vi "Out of Bounds.vi"(7 "error source vi name":string, 8 "error in (no error)":errorcluster, 9 "size":u64 format="%d bytes", 10 "offset":u64 format="%d bytes", 11 "Pointer in":refnum<class "Pointer.lvclass">) -> (0 "error out":errorcluster, 3 "Pointer out":refnum<class "Pointer.lvclass">)   [LabVIEW 2020, in "Memory Manager.lvlib" / "Pointer.lvclass"]
uses:
  Pointer.lvclass
  Errors.ctl
  VIs/Write Numeric Scalar to Source (Base10 U64).vi
  Static Errors.lvlib
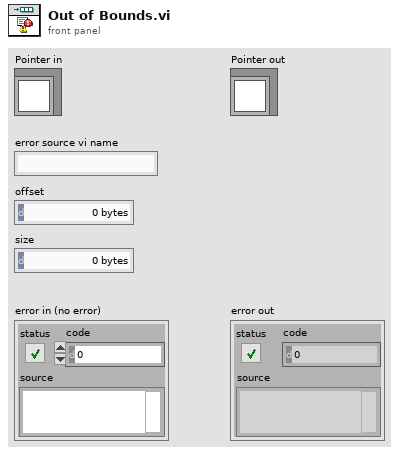
[diagram p1: front panel]
types:
  T1 = typedef "Memory Manager.lvlib/Pointer.lvclass/Errors.ctl" = enum16{"No Error", "Null Pointer", "Out of Bounds", "Buffer Underflow", "Size Mismatch", "Zone"}
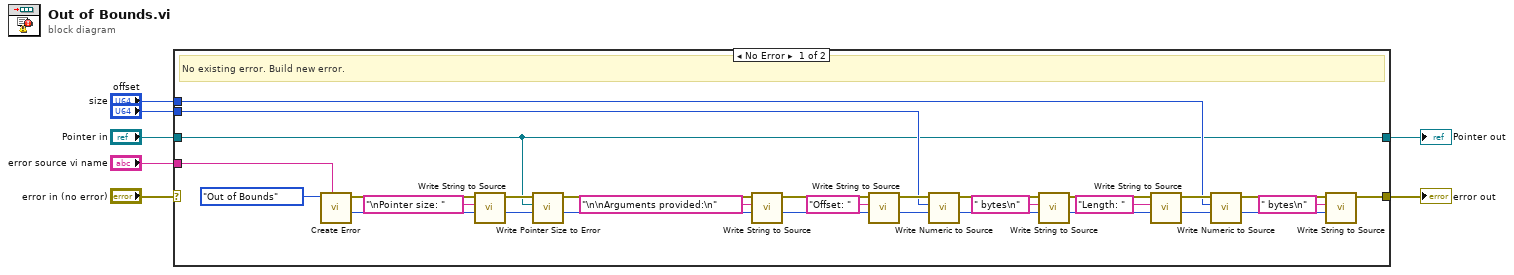
[diagram p0: block diagram]
diagram:
  n1 = case shown="No Error" "error in (no error)" {
    selector: "error in (no error)" -> [_ w39]
    tunnel: [w16 w39] -> w4
    tunnel: "offset" -> [w28 _]
    tunnel: "error source vi name" -> [w32 _]
    tunnel: "Pointer in" -> [w8 w38]
    tunnel: [w8 w38] -> w2
    tunnel: "size" -> [w15 _]
    frame No Error {
      # "No existing error. Build new error."
      n2 = call "Create Error.vi"("source vi name"=w32, "error"=Errors."Out of Bounds") -> ("new offset"=w34:i32, "error out"=w35:errorcluster)  [unwired: 8 in]
      n3 = call "Write String to Source.vi"("offset"=w34, "string"="\nPointer size: ", "error in"=w35) -> ("new offset"=w36:i32, "error out"=w9:errorcluster)  [unwired: 7 in]
      n4 = call "Write Pointer Size to Error.vi"("offset"=w36, "Pointer"=w8, "error in"=w9) -> ("new offset"=w12:i32, "error out"=w10:errorcluster)  [unwired: 7 in]
      n5 = call "Write String to Source.vi"("offset"=w12, "string"="\n\nArguments provided:\n", "error in"=w10) -> ("new offset"=w13:i32, "error out"=w14:errorcluster)  [unwired: 7 in]
      n6 = call "Write String to Source.vi"("offset"=w13, "string"="Offset: ", "error in"=w14) -> ("new offset"=w29:i32, "error out"=w30:errorcluster)  [unwired: 7 in]
      n7 = call-poly "Write Numeric to Source.vi"("offset"=w29, "value"=w28, "error in"=w30) -> ("new offset"=w25:i32, "error out"=w26:errorcluster)  [unwired: 7 in]
      n8 = call "Write String to Source.vi"("offset"=w25, "string"=" bytes\n", "error in"=w26) -> ("new offset"=w17:i32, "error out"=w18:errorcluster)  [unwired: 7 in]
      n9 = call "Write String to Source.vi"("offset"=w17, "string"="Length: ", "error in"=w18) -> ("new offset"=w22:i32, "error out"=w23:errorcluster)  [unwired: 7 in]
      n10 = call-poly "Write Numeric to Source.vi"("offset"=w22, "value"=w15, "error in"=w23) -> ("new offset"=w19:i32, "error out"=w20:errorcluster)  [unwired: 7 in]
      n11 = call "Write String to Source.vi"("offset"=w19, "string"=" bytes\n", "error in"=w20) -> ("error out"=w16:errorcluster)  [unwired: 7 in, 1 out]
    }
    frame Error {
      # "Incoming error. Pass through."
    }
  }
  "error out" <- w4
  "Pointer out" <- w2
